vi "Asylum_Driver_GetLVDTParameters.vi"(8 "error in (no error)":errorcluster, 11 "Application":refnum<k7>) -> (0 "error out":errorcluster, 2 "LVDT Parameters":T1, 3 "Application":refnum<k7>)   [LabVIEW 2019]
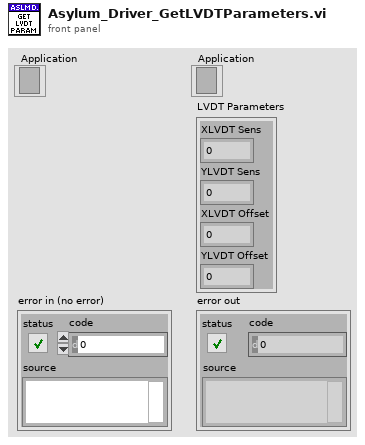
[diagram p1: front panel]
types:
  T1 = cluster{"XLVDT Sens":dbl, "YLVDT Sens":dbl, "XLVDT Offset":dbl, "YLVDT Offset":dbl}
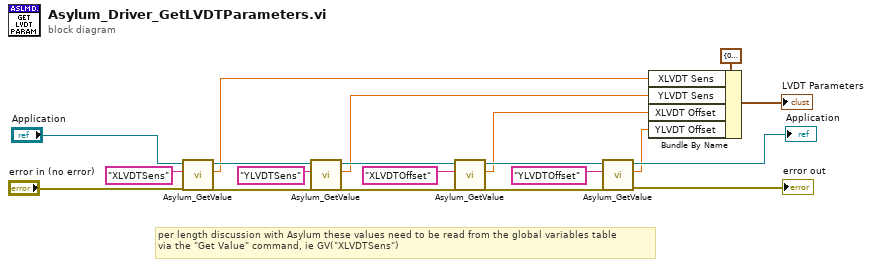
[diagram p0: block diagram]
diagram:
  # "per length discussion with Asylum these values need to be read from the global variables table\nvia the \"Get Value\" command, ie GV(\"XLVDTSens\")"
  n1 = call <userlib>:"Asylum_GetValue.vi"("error in (no error)"="error in (no error)", "Value"="XLVDTSens", "Application"="Application") -> ("error out"=w18:errorcluster, "Value"=w1:dbl, "Application"=w19:refnum<k7>)  [unwired: 6 in]
  n2 = call <userlib>:"Asylum_GetValue.vi"("error in (no error)"=w18, "Value"="YLVDTSens", "Application"=w19) -> ("error out"=w16:errorcluster, "Value"=w2:dbl, "Application"=w17:refnum<k7>)  [unwired: 6 in]
  n3 = call <userlib>:"Asylum_GetValue.vi"("error in (no error)"=w16, "Value"="XLVDTOffset", "Application"=w17) -> ("error out"=w14:errorcluster, "Value"=w3:dbl, "Application"=w15:refnum<k7>)  [unwired: 6 in]
  n4 = call <userlib>:"Asylum_GetValue.vi"("error in (no error)"=w14, "Value"="YLVDTOffset", "Application"=w15) -> ("error out"=→"error out":errorcluster, "Value"=w4:dbl, "Application"=→"Application":refnum<k7>)  [unwired: 6 in]
  n5 = Bundle By Name(cluster=T1 {"XLVDT Sens"=0.0, "YLVDT Sens"=0.0, "XLVDT Offset"=0.0, "YLVDT Offset"=0.0} ("LVDT Parameters"), "XLVDT Sens"=w1, "YLVDT Sens"=w2, "XLVDT Offset"=w3, "YLVDT Offset"=w4) -> (→"LVDT Parameters":T1)
